vi "Spectrometer.vi"(8 "error in (no error)":errorcluster, 10 "Notifiers":T1, 11 "All Message Queue Cluster":T2) -> (0 "error out":errorcluster)   [LabVIEW 2017]
doc: "Ce VI est la partie visualisation du Spectrometre. Elle permet l'envoie d'ordre à cette appareil et affiche son état.\n- Connected : indique si l'appareil est connecté.\n- Acquiring : indique si le spectrometre acquière.\n- Status : indique le status actuel du spectromètre. CAD s'il y a une erreur, ou s'il est en mouvement, etc ..."
uses:
  Lib QMH/AllMessageQueue Cluster.ctl
  Lib QMH/Message Cluster.ctl
  Lib Notifier/Notifier.ctl
  Spectro UI data.ctl
  Spectro config.ctl
  FGV Spectrometer/Action Spectro.ctl
  FGV Spectrometer/FGV Spectro Data.ctl
  Lib IHM Control/Front Panel Status.ctl
  support/Status.vi
  Lib QMH/MessageQueues.lvlib
  Lib IHM Control/IHM Control.lvlib
  Lib Notifier/Notifier.lvlib
panel:
  out "Acquiring":bool
  out "Status":string
  out "Connected":bool
  # "Spectrometer"
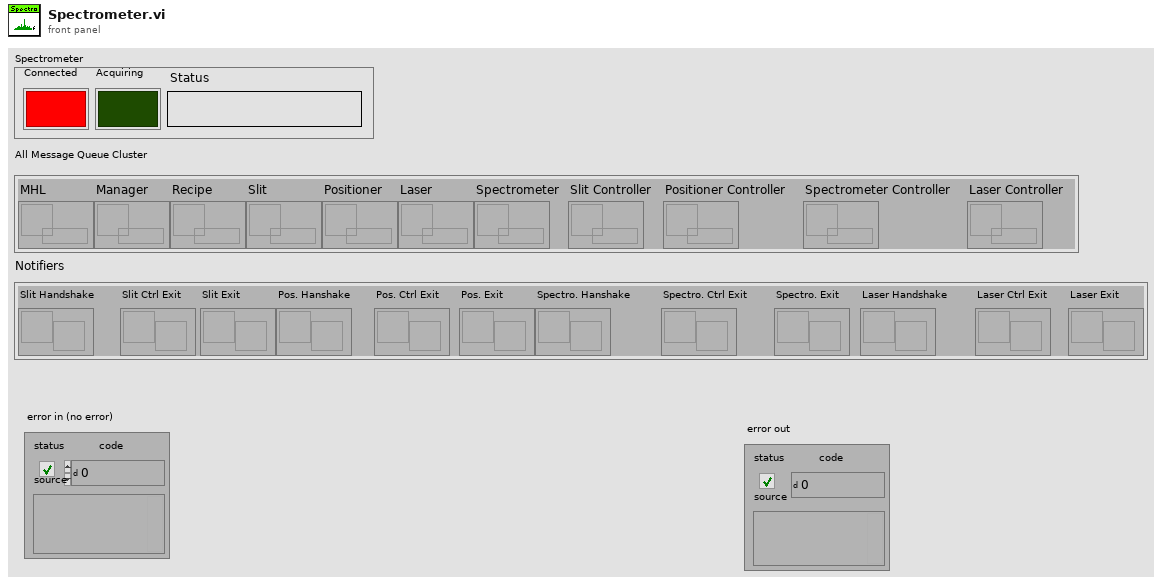
[diagram p1: front panel]
types:
  T1 = typedef "Notifier.lvlib/Notifier.ctl" = cluster{"Slit Handshake":refnum<notifier>, "Slit Ctrl Exit":refnum<notifier>, "Slit Exit":refnum<notifier>, "Pos. Hanshake":refnum<notifier>, "Pos. Ctrl Exit":refnum<notifier>, "Pos. Exit":refnum<notifier>, "Spectro. Hanshake":refnum<notifier>, "Spectro. Ctrl Exit":refnum<notifier>, "Spectro. Exit":refnum<notifier>, "Laser Handshake":refnum<notifier>, "Laser Ctrl Exit":refnum<notifier>, "Laser Exit":refnum<notifier>}
  T2 = typedef "MessageQueues.lvlib/AllMessageQueue Cluster.ctl" = cluster{"MHL":refnum<queue>, "Manager":refnum<queue>, "Recipe":refnum<queue>, "Slit":refnum<queue>, "Positioner":refnum<queue>, "Laser":refnum<queue>, "Spectrometer":refnum<queue>, "Slit Controller":refnum<queue>, "Positioner Controller":refnum<queue>, "Spectrometer Controller":refnum<queue>, "Laser Controller":refnum<queue>}
  T3 = typedef "Spectro config.ctl" = cluster{"VISA resource name":refnum<visa-resource-name>}
  T4 = typedef "Spectro UI data.ctl" = cluster{"Connected":bool, "Status":string, "Acquiring":bool}
  T5 = typedef "Action Spectro.ctl" = enum16{"Connect", "Initialisation", "Set Device", "Set Intégration time", "Get integration Time", "Disable Noise Suppress", "Enable Noise Suppress", "Set Averange", "Get Spectrum", "Get WaveLength", "Abort", "Disconnect"}
  T6 = typedef "FGV Spectro Data.ctl" = cluster{"Wrapper":u32, "Number of Spectrometers":i32, "Serial Number":string[], "Device Set":i32, "Spectre":dbl[], "Wavelength":dbl[], "Electrical Dark":enum16{"Off", "On"}, "Integration Time":i32, "Averange":i32}
  T7 = typedef "IHM Control.lvlib/Front Panel Status.ctl" = enum16{"Initialisation", "Enable Slit", "Enable Positionner", "Enable Spectrometer", "Enable Laser", "Disable Slit", "Disable Positionner", "Disable Spectrometer", "Disable Laser"}
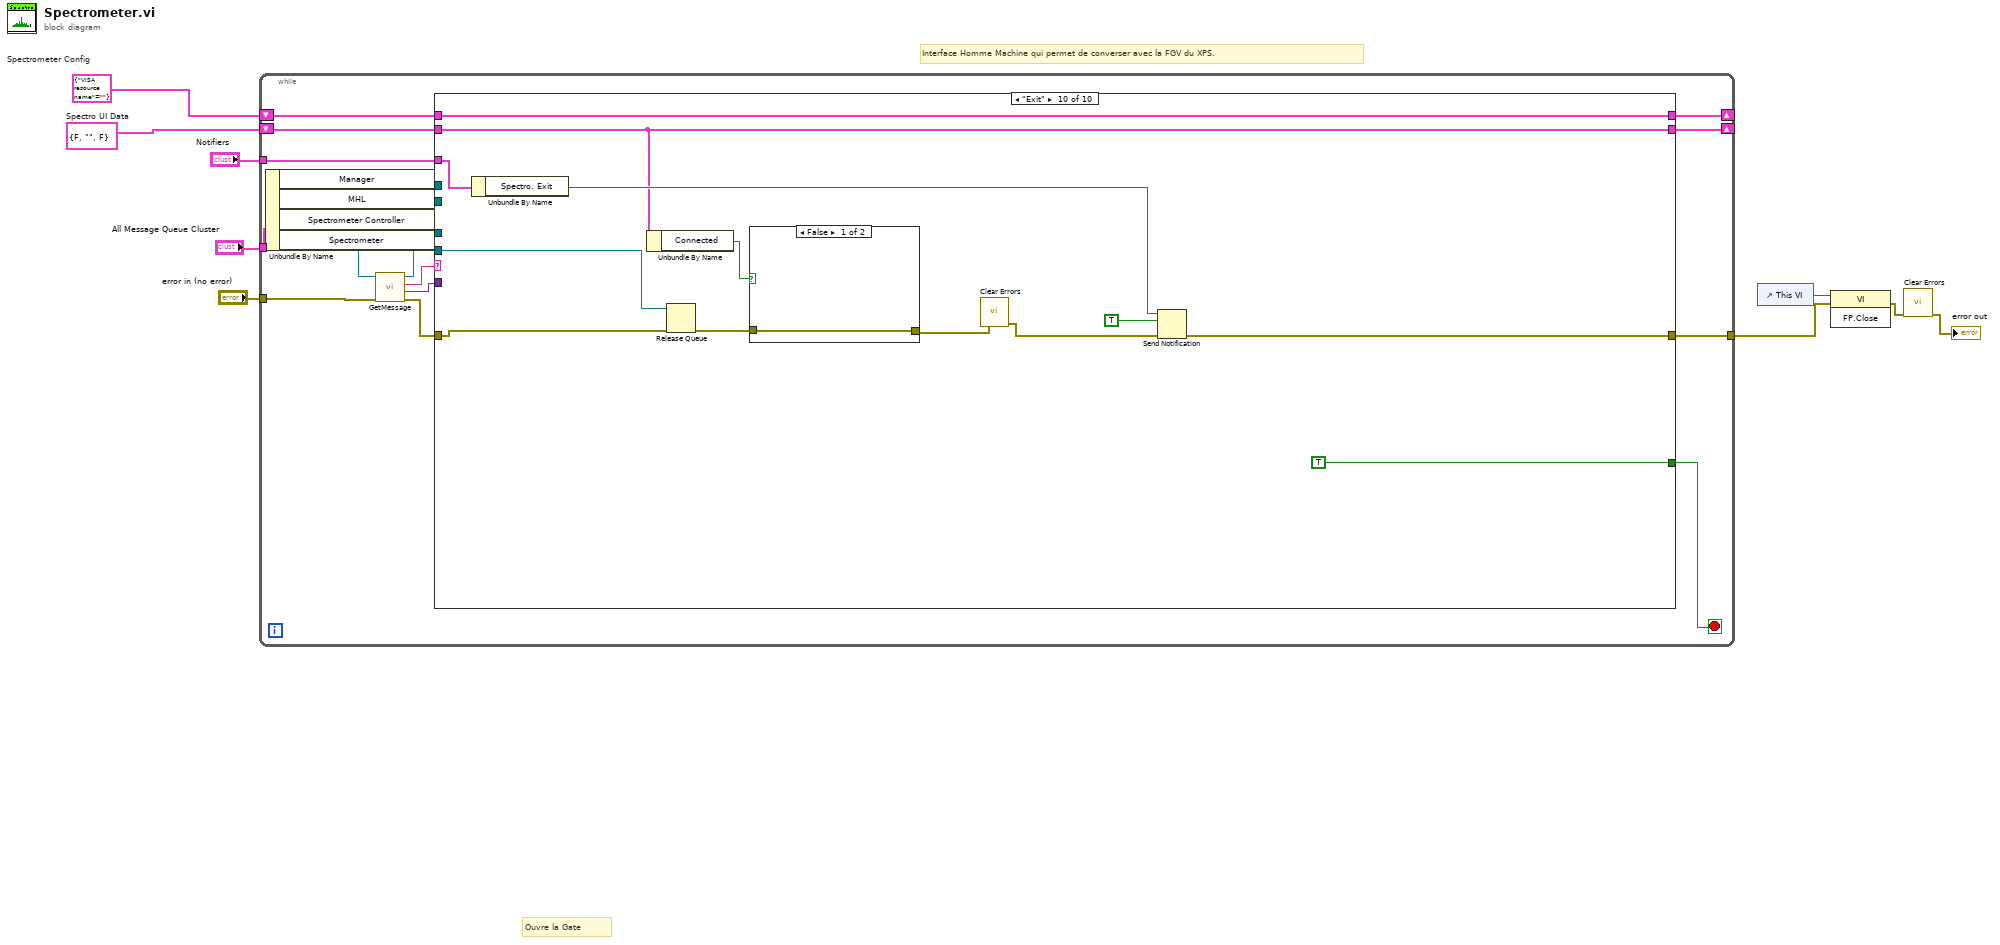
[diagram p0: block diagram]
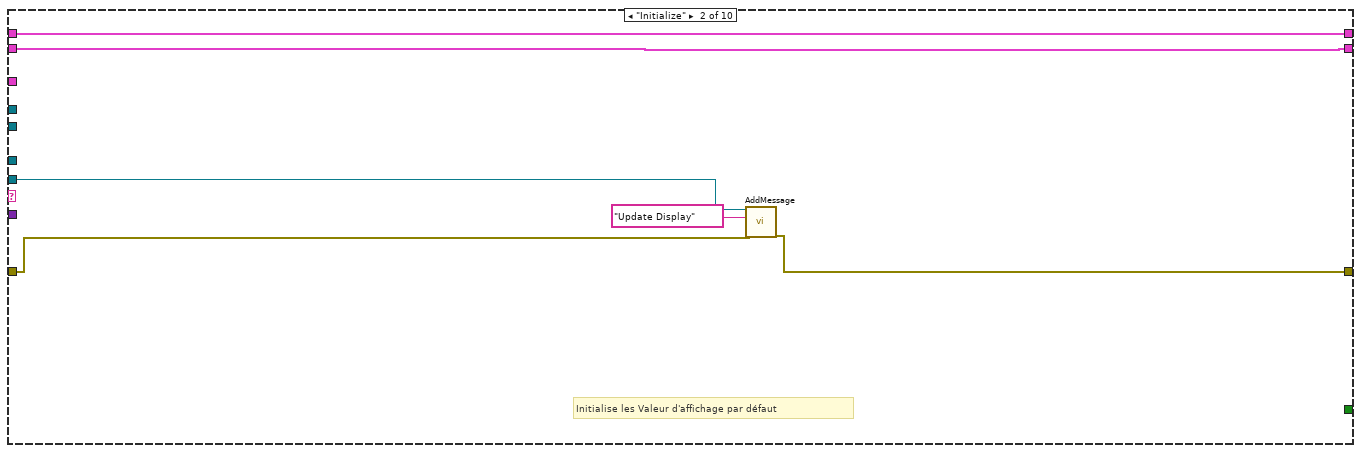
[diagram p3: hidden frame]
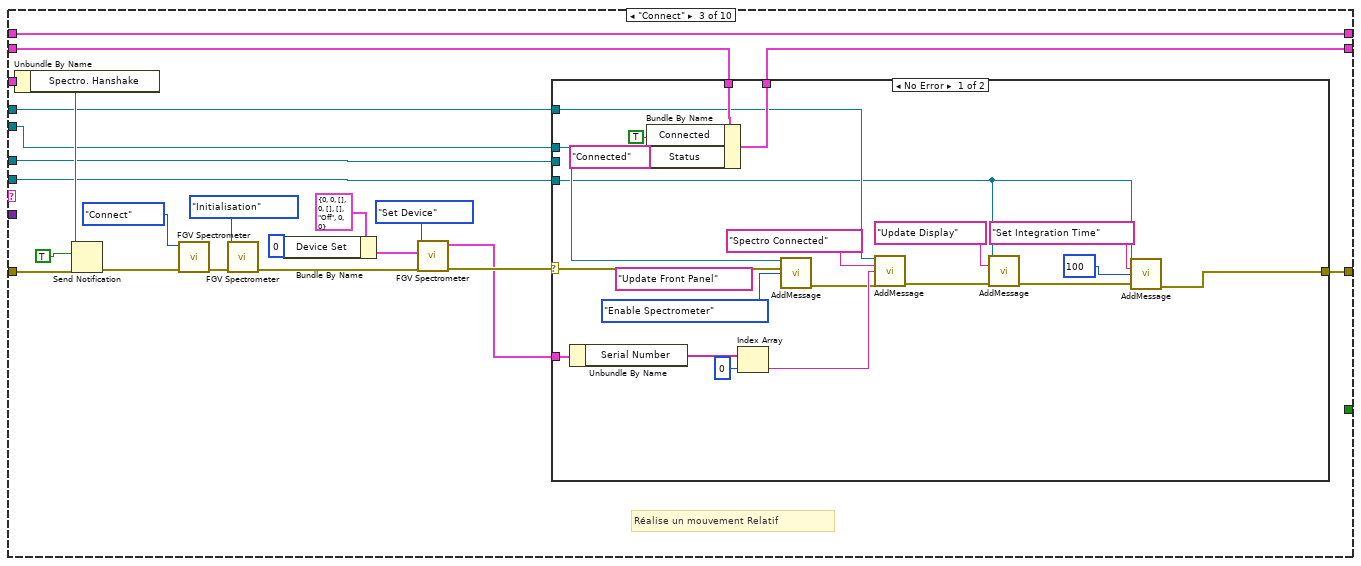
[diagram p4: hidden frame]
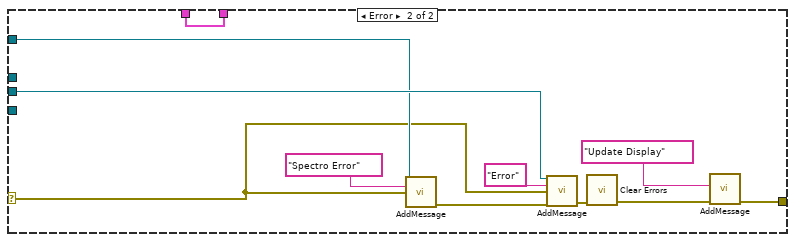
[diagram p5: hidden frame]
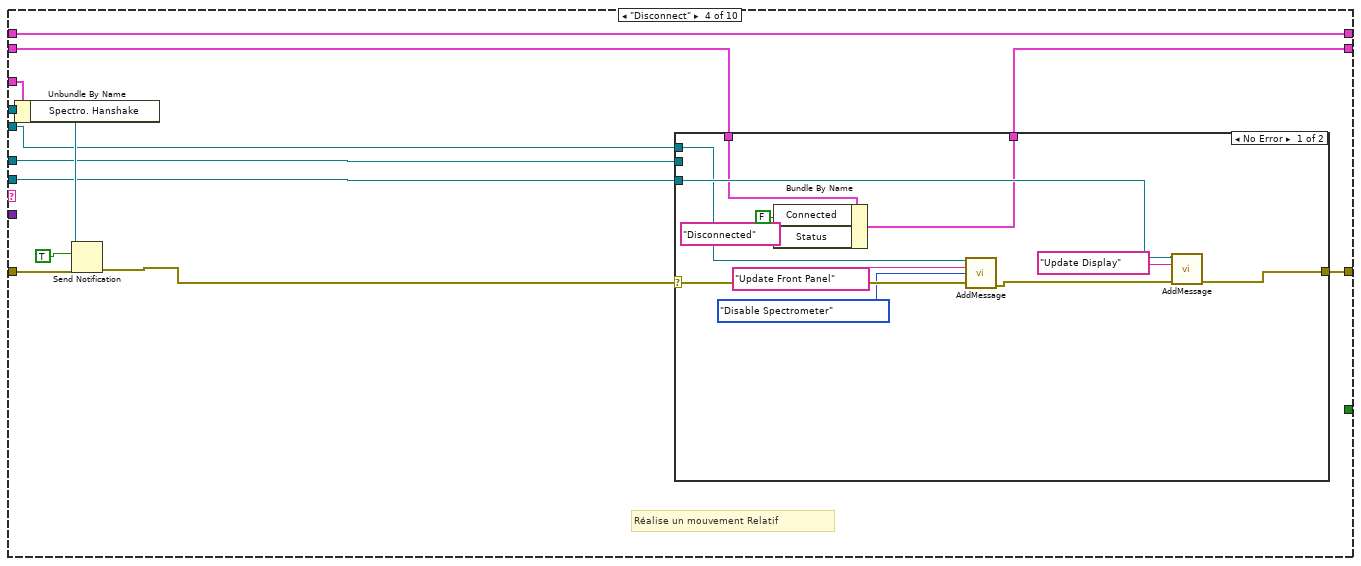
[diagram p6: hidden frame]
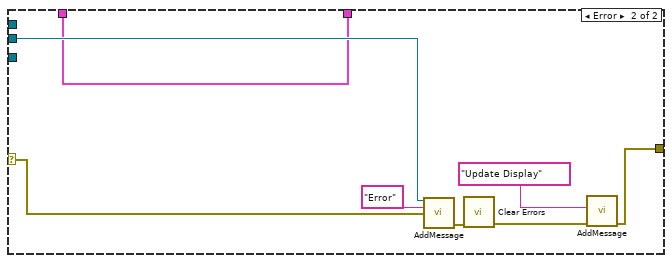
[diagram p7: hidden frame]
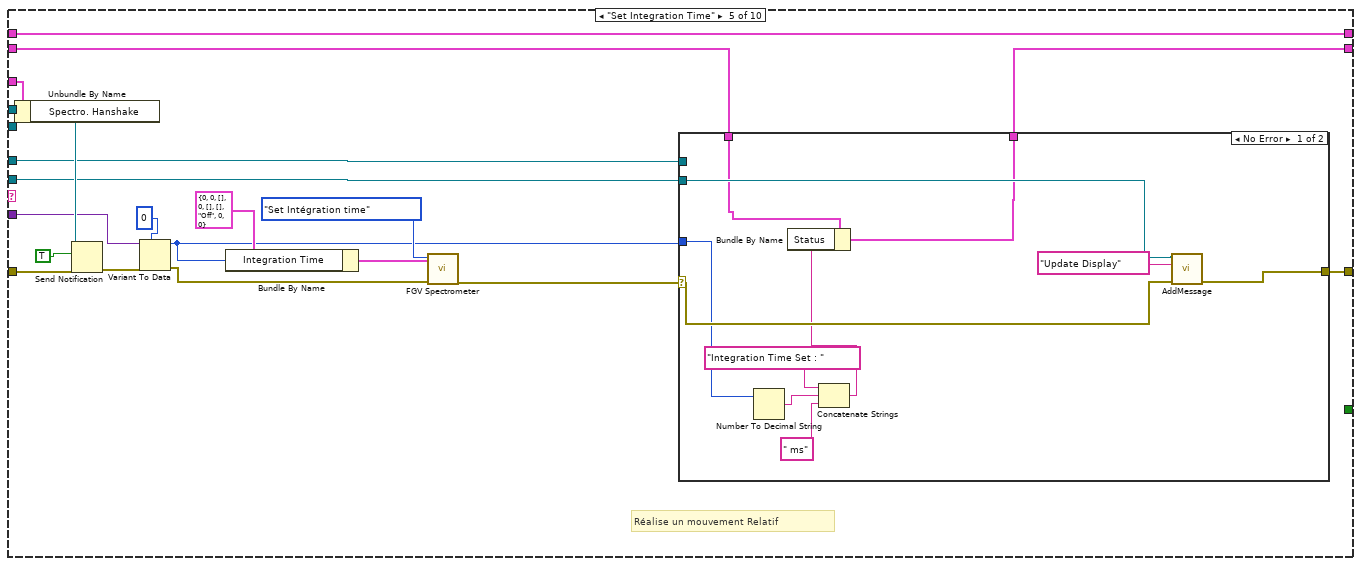
[diagram p8: hidden frame]
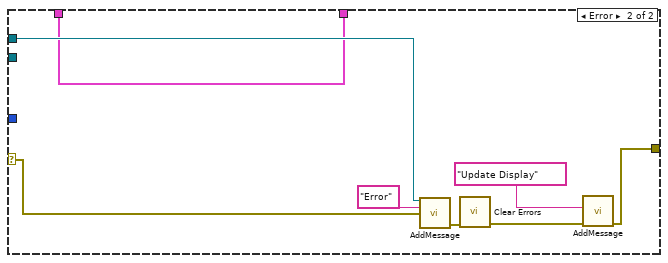
[diagram p9: hidden frame]
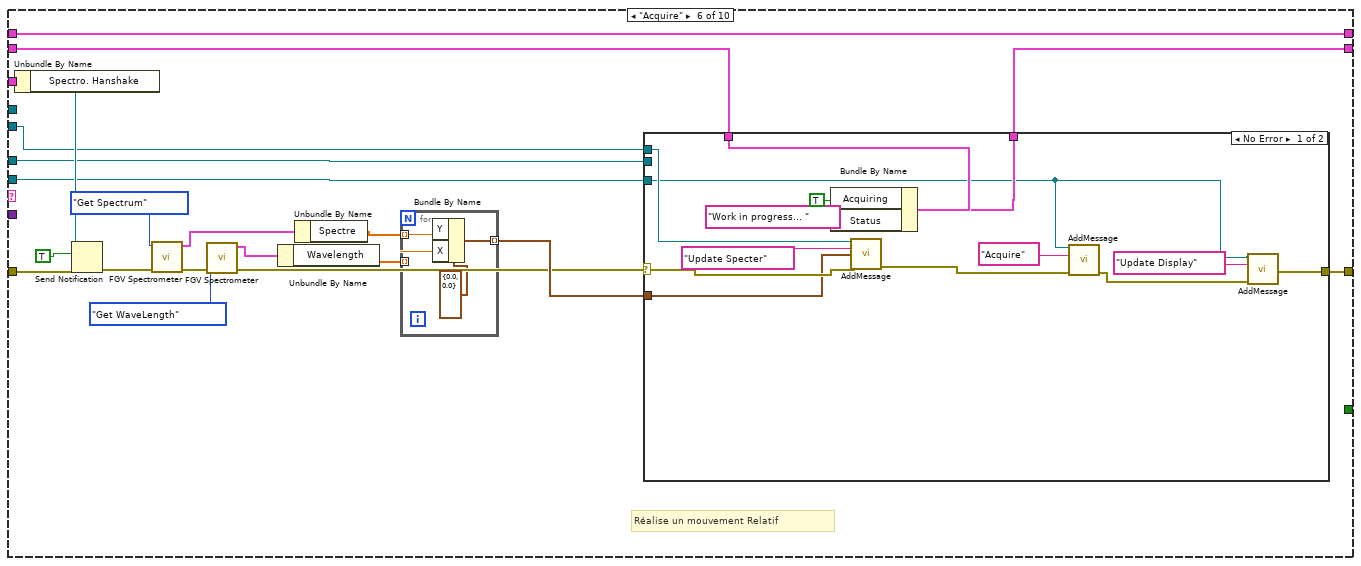
[diagram p10: hidden frame]
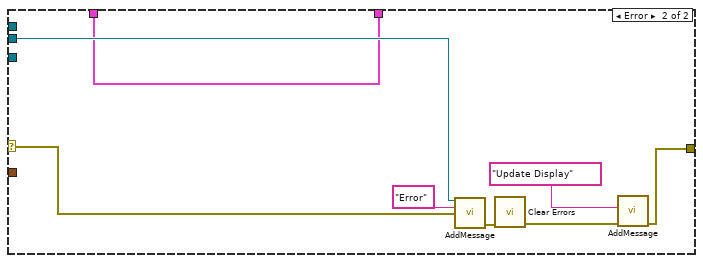
[diagram p11: hidden frame]
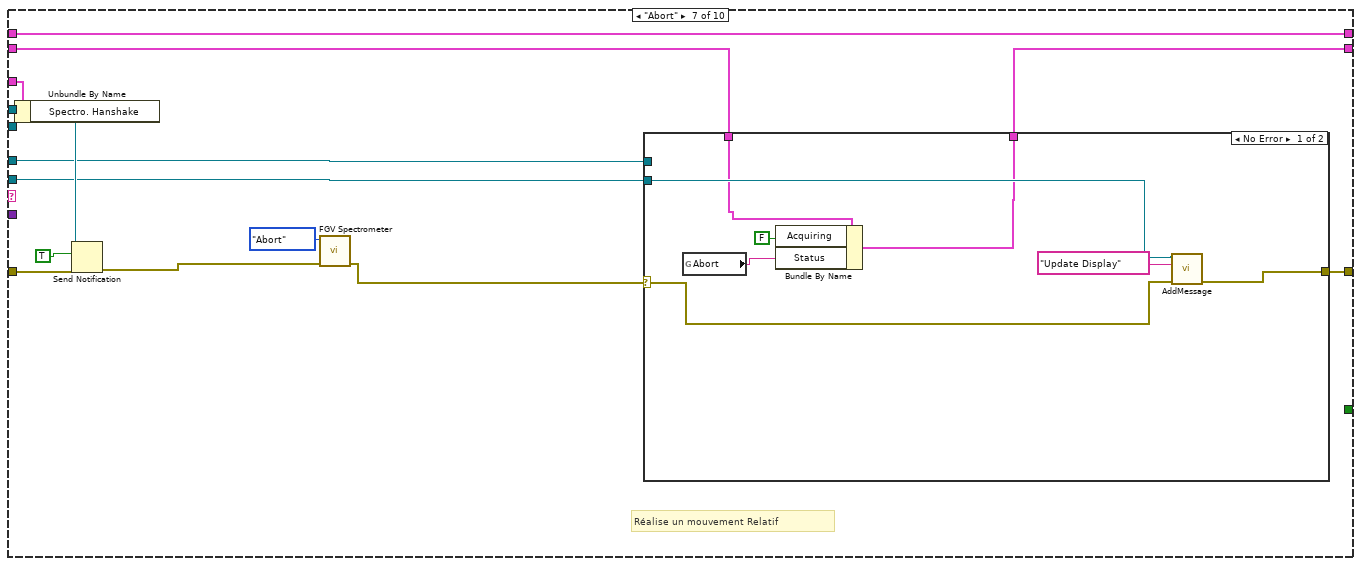
[diagram p12: hidden frame]
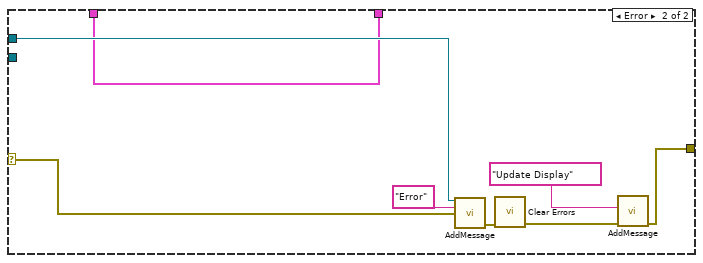
[diagram p13: hidden frame]
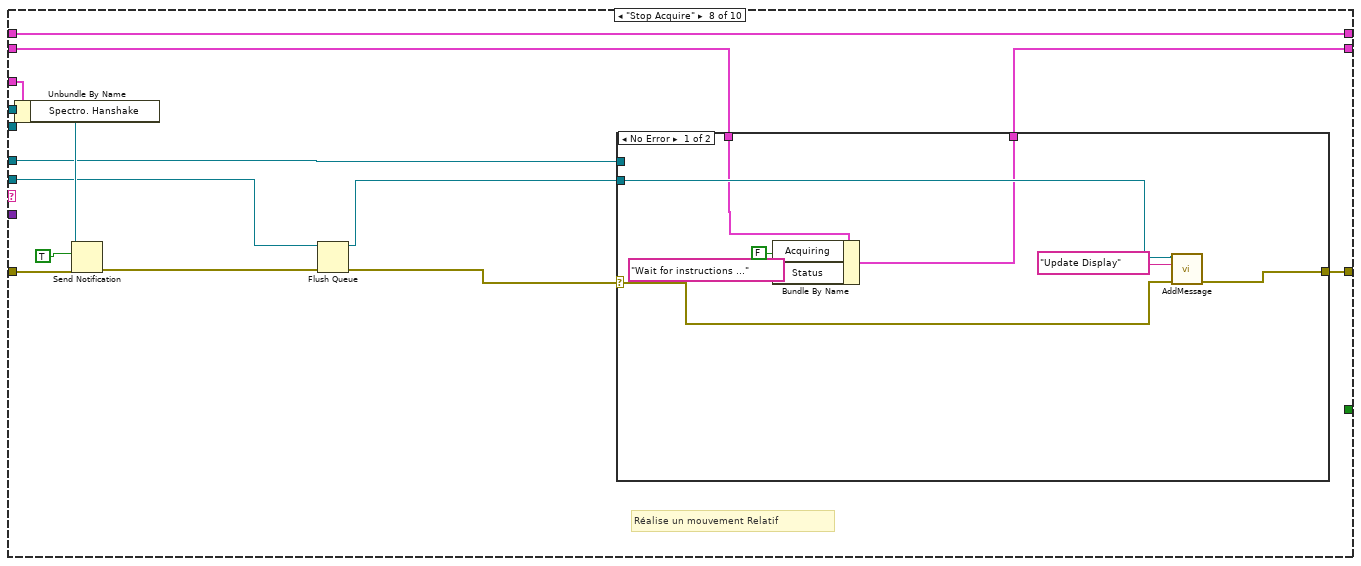
[diagram p14: hidden frame]
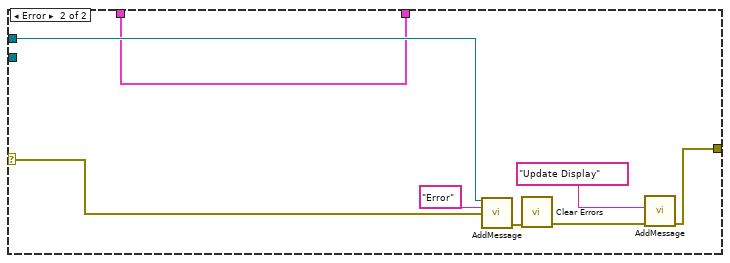
[diagram p15: hidden frame]
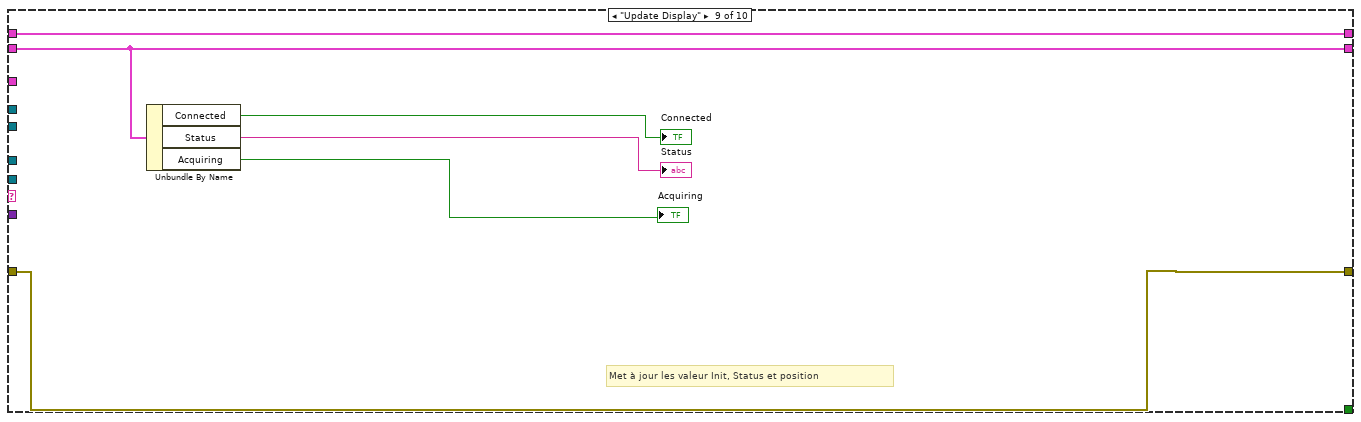
[diagram p16: hidden frame]
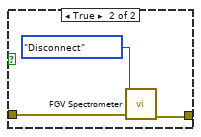
[diagram p17: hidden frame]
diagram:
  w5 = T3 {"VISA resource name"=""}  # Spectrometer Config
  w6 = T4 {"Connected"=FALSE, "Status"="", "Acquiring"=FALSE}  # Spectro UI Data
  # "Interface Homme Machine qui permet de converser avec la FGV du XPS."
  # "Ouvre la Gate"
  n1 = while {
    tunnel: "All Message Queue Cluster" -> [w20]
    tunnel: "Notifiers" -> [w26]
    tunnel: "error in (no error)" -> [w21]
    tunnel: [w19] -> w2
    shift-right: [w15] -> _
    shift-left: w5 -> [w16]
    shift-right: [w13] -> _
    shift-left: w6 -> [w14]
    stop <- w17 stop-if-true
    n2 = Unbundle By Name(w20) -> ("Manager"=w10:refnum<queue>, "MHL"=w11:refnum<queue>, "Spectrometer Controller"=w18:refnum<queue>, "Spectrometer"=w12:refnum<queue>)
    n3 = call "GetMessage.vi"("entrée d'erreur"=w21, "Message queue"=w12) -> ("sortie d'erreur"=w22:errorcluster, "Data"=w23:variant, "Message"=w24:string, "Dup Message Queue"=w25:refnum<queue>)  [unwired: 6 in]
    n4 = case shown="\"Exit\"" w24 {
      tunnel: w26 -> [_ _ w56 w101 w140 w180 w219 w248 _ w284]
      tunnel: w25 -> [_ w30 w55 w100 w139 w179 w218 w239 _ w278]
      tunnel: w23 -> [_ _ _ _ w131 _ _ _ _ _]
      tunnel: w22 -> [w29 w33 w49 w94 w133 w173 w212 w242 w271 w279]
      tunnel: [w29 w32 w54 w99 w138 w178 w217 w247 w271 w281] -> w19
      tunnel: w18 -> [_ _ w53 w98 w137 w177 w216 w246 _ _]
      tunnel: [_ _ _ _ _ _ _ _ _ TRUE] -> w17
      tunnel: w16 -> [w28 w35 w52 w97 w136 w176 w215 w245 w272 w280]
      tunnel: [w28 w35 w52 w97 w136 w176 w215 w245 w272 w280] -> w15
      tunnel: w14 -> [w27 w31 w51 w96 w135 w175 w214 w244 w270 w274]
      tunnel: [w27 w31 w50 w95 w134 w174 w213 w243 w270 w274] -> w13
      tunnel: w11 -> [_ _ w48 w93 _ w170 _ _ _ _]
      tunnel: w10 -> [_ _ w47 _ _ _ _ _ _ _]
      frame Default {
        # "ne fait rien si le message dépilé n'existe pas"
      }
      frame "Initialize" {
        # "Initialise les Valeur d'affichage par défaut"
        n5 = call "AddMessage.vi"("Message queue"=w30, "Message"="Update Display", "entrée d'erreur (pas d'erreur)"=w33) -> ("error out"=w32:errorcluster)  [unwired: 11 in, 1 out]
      }
      frame "Connect" {
        # "Réalise un mouvement Relatif"
        n6 = Unbundle By Name(w56) -> ("Spectro. Hanshake"=w58:refnum<notifier>)
        n7 = Send Notification(notification=TRUE, notifier=w58, error in (no error)=w49) -> (error out=w46:errorcluster)  [unwired: 1 out]
        n8 = call "FGV Spectrometer.vi"("entrée d'erreur (pas d'erreur)"=w46, "Action"=Action_Spectro."Connect") -> ("sortie d'erreur"=w43:errorcluster)  [unwired: 8 in, 1 out]
        n9 = call "FGV Spectrometer.vi"("entrée d'erreur (pas d'erreur)"=w43, "Action"=Action_Spectro."Initialisation") -> ("sortie d'erreur"=w42:errorcluster)  [unwired: 8 in, 1 out]
        n10 = Bundle By Name(cluster=T6 {"Wrapper"=0, "Number of Spectrometers"=0, "Serial Number"=[], "Device Set"=0, "Spectre"=[], "Wavelength"=[], "Electrical Dark"=enum."Off", "Integration Time"=0, "Averange"=0} ("FGV Spectrometer Data"), "Device Set"=0) -> (w38:T6)
        n11 = call "FGV Spectrometer.vi"("entrée d'erreur (pas d'erreur)"=w42, "FGV Spectro. Data"=w38, "Action"=Action_Spectro."Set Device") -> ("sortie d'erreur"=w41:errorcluster, "Data out"=w36:T6)  [unwired: 7 in]
        n12 = case shown="No Error" w41 {
          selector: w41 -> [w76 w82]
          tunnel: w55 -> [w61 _]
          tunnel: [w62 w87] -> w54
          tunnel: w53 -> [_ w86]
          tunnel: w51 -> [w79 w85]
          tunnel: [w78 w85] -> w50
          tunnel: w48 -> [w66 _]
          tunnel: w47 -> [w73 w83]
          tunnel: w36 -> [w70 _]
          frame No Error {
            n13 = Unbundle By Name(w70) -> ("Serial Number"=w69:string[])
            n14 = Bundle By Name(cluster=w79, "Connected"=TRUE, "Status"="Connected") -> (w78:T4)
            n15 = Index Array(array=w69, index=0) -> (element=w67:string)
            n16 = call "AddMessage.vi"("Message queue"=w66, "Message"="Update Front Panel", "Data"=Front_Panel_Status."Enable Spectrometer" ("Front Panel status"), "entrée d'erreur (pas d'erreur)"=w76) -> ("error out"=w65:errorcluster)  [unwired: 10 in, 1 out]
            n17 = call "AddMessage.vi"("Message queue"=w73, "Message"="Spectro Connected", "Data"=w67, "entrée d'erreur (pas d'erreur)"=w65) -> ("error out"=w64:errorcluster)  [unwired: 10 in, 1 out]
            n18 = call "AddMessage.vi"("Message queue"=w61, "Message"="Update Display", "entrée d'erreur (pas d'erreur)"=w64) -> ("error out"=w63:errorcluster)  [unwired: 11 in, 1 out]
            n19 = call "AddMessage.vi"("Message queue"=w61, "Message"="Set Integration Time", "Data"=100 ("index"), "entrée d'erreur (pas d'erreur)"=w63) -> ("error out"=w62:errorcluster)  [unwired: 10 in, 1 out]
          }
          frame Error {
            n20 = call "AddMessage.vi"("Message queue"=w83, "Message"="Spectro Error", "Data"=w82) -> ("error out"=w81:errorcluster)  [unwired: 11 in, 1 out]
            n21 = call "AddMessage.vi"("Message queue"=w86, "Message"="Error", "Data"=w82, "entrée d'erreur (pas d'erreur)"=w81) -> ("error out"=w90:errorcluster)  [unwired: 10 in, 1 out]
            n22 = call <vilib>:"Clear Errors.vi"("error in (no error)"=w90) -> ("error out"=w88:errorcluster)  [unwired: 5 in, 1 out]
            n23 = call "AddMessage.vi"("Message"="Update Display", "entrée d'erreur (pas d'erreur)"=w88) -> ("error out"=w87:errorcluster)  [unwired: 12 in, 1 out]
          }
        }
      }
      frame "Disconnect" {
        # "Réalise un mouvement Relatif"
        n24 = Unbundle By Name(w101) -> ("Spectro. Hanshake"=w103:refnum<notifier>)
        n25 = Send Notification(notification=TRUE, notifier=w103, error in (no error)=w94) -> (error out=w92:errorcluster)  [unwired: 1 out]
        n26 = case shown="No Error" w92 {
          selector: w92 -> [w109 w118]
          tunnel: w100 -> [w115 _]
          tunnel: [w113 w119] -> w99
          tunnel: w98 -> [_ w117]
          tunnel: w96 -> [w112 w116]
          tunnel: [w111 w116] -> w95
          tunnel: w93 -> [w107 _]
          frame No Error {
            n27 = Bundle By Name(cluster=w112, "Connected"=FALSE, "Status"="Disconnected") -> (w111:T4)
            n28 = call "AddMessage.vi"("Message queue"=w107, "Message"="Update Front Panel", "Data"=Front_Panel_Status."Disable Spectrometer" ("Front Panel status"), "entrée d'erreur (pas d'erreur)"=w109) -> ("error out"=w108:errorcluster)  [unwired: 10 in, 1 out]
            n29 = call "AddMessage.vi"("Message queue"=w115, "Message"="Update Display", "entrée d'erreur (pas d'erreur)"=w108) -> ("error out"=w113:errorcluster)  [unwired: 11 in, 1 out]
          }
          frame Error {
            n30 = call "AddMessage.vi"("Message queue"=w117, "Message"="Error", "Data"=w118) -> ("error out"=w122:errorcluster)  [unwired: 11 in, 1 out]
            n31 = call <vilib>:"Clear Errors.vi"("error in (no error)"=w122) -> ("error out"=w120:errorcluster)  [unwired: 5 in, 1 out]
            n32 = call "AddMessage.vi"("Message"="Update Display", "entrée d'erreur (pas d'erreur)"=w120) -> ("error out"=w119:errorcluster)  [unwired: 12 in, 1 out]
          }
        }
      }
      frame "Set Integration Time" {
        # "Réalise un mouvement Relatif"
        n33 = Unbundle By Name(w140) -> ("Spectro. Hanshake"=w142:refnum<notifier>)
        n34 = Send Notification(notification=TRUE, notifier=w142, error in (no error)=w133) -> (error out=w132:errorcluster)  [unwired: 1 out]
        n35 = Variant To Data(error in=w132, type=0, Variant=w131) -> (data=w124:i32, error out=w129:errorcluster)
        n36 = Bundle By Name(cluster=T6 {"Wrapper"=0, "Number of Spectrometers"=0, "Serial Number"=[], "Device Set"=0, "Spectre"=[], "Wavelength"=[], "Electrical Dark"=enum."Off", "Integration Time"=0, "Averange"=0} ("FGV Spectrometer Data"), "Integration Time"=w124) -> (w126:T6)
        n37 = call "FGV Spectrometer.vi"("entrée d'erreur (pas d'erreur)"=w129, "FGV Spectro. Data"=w126, "Action"=Action_Spectro."Set Intégration time") -> ("sortie d'erreur"=w128:errorcluster)  [unwired: 7 in, 1 out]
        n38 = case shown="No Error" w128 {
          selector: w128 -> [w150 w156]
          tunnel: w139 -> [w153 _]
          tunnel: [w151 w157] -> w138
          tunnel: w137 -> [_ w155]
          tunnel: w135 -> [w149 w154]
          tunnel: [w148 w154] -> w134
          tunnel: w124 -> [w143 _]
          frame No Error {
            n39 = Number To Decimal String(number=w143) -> (decimal integer string=w146:string)  [unwired: 1 in]
            n40 = Concatenate Strings("Integration Time Set : " ("string"), w146, " ms" ("string")) -> (w144:string)
            n41 = Bundle By Name(cluster=w149, "Status"=w144) -> (w148:T4)
            n42 = call "AddMessage.vi"("Message queue"=w153, "Message"="Update Display", "entrée d'erreur (pas d'erreur)"=w150) -> ("error out"=w151:errorcluster)  [unwired: 11 in, 1 out]
          }
          frame Error {
            n43 = call "AddMessage.vi"("Message queue"=w155, "Message"="Error", "Data"=w156) -> ("error out"=w160:errorcluster)  [unwired: 11 in, 1 out]
            n44 = call <vilib>:"Clear Errors.vi"("error in (no error)"=w160) -> ("error out"=w158:errorcluster)  [unwired: 5 in, 1 out]
            n45 = call "AddMessage.vi"("Message"="Update Display", "entrée d'erreur (pas d'erreur)"=w158) -> ("error out"=w157:errorcluster)  [unwired: 12 in, 1 out]
          }
        }
      }
      frame "Acquire" {
        # "Réalise un mouvement Relatif"
        n46 = Unbundle By Name(w180) -> ("Spectro. Hanshake"=w182:refnum<notifier>)
        n47 = Send Notification(notification=TRUE, notifier=w182, error in (no error)=w173) -> (error out=w172:errorcluster)  [unwired: 1 out]
        n48 = call "FGV Spectrometer.vi"("entrée d'erreur (pas d'erreur)"=w172, "Action"=Action_Spectro."Get Spectrum") -> ("sortie d'erreur"=w164:errorcluster, "Data out"=w166:T6)  [unwired: 8 in]
        n49 = call "FGV Spectrometer.vi"("entrée d'erreur (pas d'erreur)"=w164, "Action"=Action_Spectro."Get WaveLength") -> ("sortie d'erreur"=w163:errorcluster, "Data out"=w167:T6)  [unwired: 8 in]
        n50 = Unbundle By Name(w167) -> ("Wavelength"=w169:dbl[])
        n51 = Unbundle By Name(w166) -> ("Spectre"=w165:dbl[])
        n52 = for {
          tunnel: w165 -> [w183] mode=indexing
          tunnel: w169 -> [w184] mode=indexing
          tunnel: [w185] -> w168 mode=indexing
          n53 = Bundle By Name(cluster=cluster{"X":dbl, "Y":dbl} {"X"=0.0, "Y"=0.0}, "Y"=w183, "X"=w184) -> (w185:cluster{"X":dbl, "Y":dbl})
        }
        n54 = case shown="No Error" w163 {
          selector: w163 -> [w191 w203]
          tunnel: w179 -> [w188 _]
          tunnel: [w199 w204] -> w178
          tunnel: w177 -> [_ w202]
          tunnel: w175 -> [w197 w201]
          tunnel: [w196 w201] -> w174
          tunnel: w170 -> [w192 _]
          tunnel: w168 -> [w187 _]
          frame No Error {
            n55 = Bundle By Name(cluster=w197, "Acquiring"=TRUE ("Connected"), "Status"="Work in progress... ") -> (w196:T4)
            n56 = call "AddMessage.vi"("Message queue"=w192, "Message"="Update Specter", "Data"=w187, "entrée d'erreur (pas d'erreur)"=w191) -> ("error out"=w190:errorcluster)  [unwired: 10 in, 1 out]
            n57 = call "AddMessage.vi"("Message queue"=w188, "Message"="Acquire", "entrée d'erreur (pas d'erreur)"=w190) -> ("error out"=w189:errorcluster)  [unwired: 11 in, 1 out]
            n58 = call "AddMessage.vi"("Message queue"=w188, "Message"="Update Display", "entrée d'erreur (pas d'erreur)"=w189) -> ("error out"=w199:errorcluster)  [unwired: 11 in, 1 out]
          }
          frame Error {
            n59 = call "AddMessage.vi"("Message queue"=w202, "Message"="Error", "Data"=w203) -> ("error out"=w207:errorcluster)  [unwired: 11 in, 1 out]
            n60 = call <vilib>:"Clear Errors.vi"("error in (no error)"=w207) -> ("error out"=w205:errorcluster)  [unwired: 5 in, 1 out]
            n61 = call "AddMessage.vi"("Message"="Update Display", "entrée d'erreur (pas d'erreur)"=w205) -> ("error out"=w204:errorcluster)  [unwired: 12 in, 1 out]
          }
        }
      }
      frame "Abort" {
        # "Réalise un mouvement Relatif"
        n62 = Unbundle By Name(w219) -> ("Spectro. Hanshake"=w221:refnum<notifier>)
        n63 = Send Notification(notification=TRUE, notifier=w221, error in (no error)=w212) -> (error out=w211:errorcluster)  [unwired: 1 out]
        n64 = call "FGV Spectrometer.vi"("entrée d'erreur (pas d'erreur)"=w211, "Action"=Action_Spectro."Abort") -> ("sortie d'erreur"=w210:errorcluster)  [unwired: 8 in, 1 out]
        n65 = case shown="No Error" w210 {
          selector: w210 -> [w226 w232]
          tunnel: w218 -> [w229 _]
          tunnel: [w227 w233] -> w217
          tunnel: w216 -> [_ w231]
          tunnel: w214 -> [w224 w230]
          tunnel: [w223 w230] -> w213
          frame No Error {
            n66 = global read "Status.vi" "Abort"() -> (w222:string)
            n67 = Bundle By Name(cluster=w224, "Acquiring"=FALSE ("Connected"), "Status"=w222) -> (w223:T4)
            n68 = call "AddMessage.vi"("Message queue"=w229, "Message"="Update Display", "entrée d'erreur (pas d'erreur)"=w226) -> ("error out"=w227:errorcluster)  [unwired: 11 in, 1 out]
          }
          frame Error {
            n69 = call "AddMessage.vi"("Message queue"=w231, "Message"="Error", "Data"=w232) -> ("error out"=w236:errorcluster)  [unwired: 11 in, 1 out]
            n70 = call <vilib>:"Clear Errors.vi"("error in (no error)"=w236) -> ("error out"=w234:errorcluster)  [unwired: 5 in, 1 out]
            n71 = call "AddMessage.vi"("Message"="Update Display", "entrée d'erreur (pas d'erreur)"=w234) -> ("error out"=w233:errorcluster)  [unwired: 12 in, 1 out]
          }
        }
      }
      frame "Stop Acquire" {
        # "Réalise un mouvement Relatif"
        n72 = Unbundle By Name(w248) -> ("Spectro. Hanshake"=w250:refnum<notifier>)
        n73 = Send Notification(notification=TRUE, notifier=w250, error in (no error)=w242) -> (error out=w241:errorcluster)  [unwired: 1 out]
        n74 = Flush Queue(queue=w239, error in (no error)=w241) -> (queue out=w238:refnum<queue>, error out=w240:errorcluster)  [unwired: 1 out]
        n75 = case shown="No Error" w240 {
          selector: w240 -> [w255 w261]
          tunnel: w238 -> [w258 _]
          tunnel: [w256 w262] -> w247
          tunnel: w246 -> [_ w260]
          tunnel: w244 -> [w253 w259]
          tunnel: [w252 w259] -> w243
          frame No Error {
            n76 = Bundle By Name(cluster=w253, "Acquiring"=FALSE ("Connected"), "Status"="Wait for instructions ...") -> (w252:T4)
            n77 = call "AddMessage.vi"("Message queue"=w258, "Message"="Update Display", "entrée d'erreur (pas d'erreur)"=w255) -> ("error out"=w256:errorcluster)  [unwired: 11 in, 1 out]
          }
          frame Error {
            n78 = call "AddMessage.vi"("Message queue"=w260, "Message"="Error", "Data"=w261) -> ("error out"=w265:errorcluster)  [unwired: 11 in, 1 out]
            n79 = call <vilib>:"Clear Errors.vi"("error in (no error)"=w265) -> ("error out"=w263:errorcluster)  [unwired: 5 in, 1 out]
            n80 = call "AddMessage.vi"("Message"="Update Display", "entrée d'erreur (pas d'erreur)"=w263) -> ("error out"=w262:errorcluster)  [unwired: 12 in, 1 out]
          }
        }
      }
      frame "Update Display" {
        # "Met à jour les valeur Init, Status et position"
        n81 = Unbundle By Name(w270) -> ("Connected"=→"Connected":bool, "Status"=→"Status":string, "Acquiring"=→"Acquiring":bool)
      }
      frame "Exit" {
        n82 = Unbundle By Name(w284) -> ("Spectro. Exit"=w283:refnum<notifier>)
        n83 = Unbundle By Name(w274) -> ("Connected"=w273:bool)
        n84 = Release Queue(queue=w278, error in (no error)=w279) -> (error out=w277:errorcluster)  [unwired: 1 in, 2 out]
        n85 = case shown="False" w273 {
          tunnel: w277 -> [w286 w289]
          tunnel: [w286 w288] -> w276
          frame False {
          }
          frame True {
            n86 = call "FGV Spectrometer.vi"("entrée d'erreur (pas d'erreur)"=w289, "Action"=Action_Spectro."Disconnect") -> ("sortie d'erreur"=w288:errorcluster)  [unwired: 8 in, 1 out]
          }
        }
        n87 = call <vilib>:"Clear Errors.vi"("error in (no error)"=w276) -> ("error out"=w275:errorcluster)  [unwired: 5 in, 1 out]
        n88 = Send Notification(notification=TRUE, notifier=w283, error in (no error)=w275) -> (error out=w281:errorcluster)  [unwired: 1 out]
      }
    }
  }
  n89 = control-ref of="This VI"() -> (w4:refnum<vi>)
  n90 = invoke class="VI" method="FP.Close"(reference=w4, error in=w2) -> (error out=w3:errorcluster)  [unwired: 1 in, 2 out]
  n91 = call <vilib>:"Clear Errors.vi"("error in (no error)"=w3) -> ("error out"=→"error out":errorcluster)  [unwired: 5 in, 1 out]
